vi "Sst To Dkm.vi"(8 "error in (no error)":errorcluster, 10 "error":i32, 11 "sStations":string) -> (0 "error out":i32, 1 "error out 2":errorcluster, 2 "dkm":dbl, 3 "sStations out":string)   [LabVIEW 2023, in "POSCONV.lvlib"]
doc: "Converts string stations into double kilometres (One station is 100 ft = 0.03048 km)...\n\ndouble SstToDkm(char *sStations, int *error);"
uses:
  POSCONV.lvlib
  C:/Users/J Gordon/Documents/Rail Tech/TV-HR/02 - Code/Modules/POSCONV/POSCONV.dll
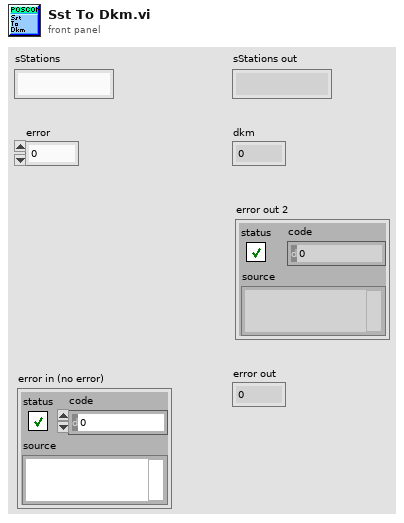
[diagram p1: front panel]
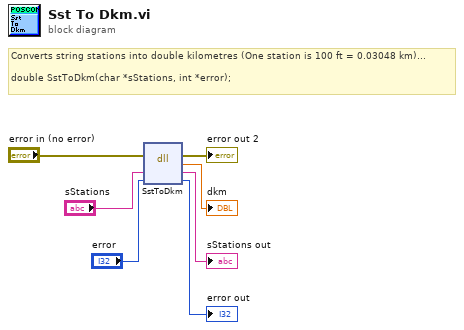
[diagram p0: block diagram]
diagram:
  # "Converts string stations into double kilometres (One station is 100 ft = 0.03048 km)...\n\ndouble SstToDkm(char *sStations, int *error);"
  n1 = dll-call lib="C:/Users/J Gordon/Documents/Rail Tech/TV-HR/02 - Code/Modules/POSCONV/POSCONV.*" fn="SstToDkm"(error in="error in (no error)", "sStations"="sStations", "error"="error") -> (error out=→"error out 2":errorcluster, →"dkm":dbl, "sStations"=→"sStations out":string, "error"=→"error out":i32)  [unwired: 2 in, 1 out]
